vi "GetPen.vi"(8 "error in (no error)":errorcluster, 11 "Pen in":refnum<class "Pen.lvclass">) -> (0 "error out":errorcluster, 2 "Pen":T1, 3 "Pen out":refnum<class "Pen.lvclass">)   [LabVIEW 2021, in "Picture2D.lvlib" / "Pen.lvclass"]
uses:
  Pen.lvclass
  Pen.lvclass/Pen.ctl
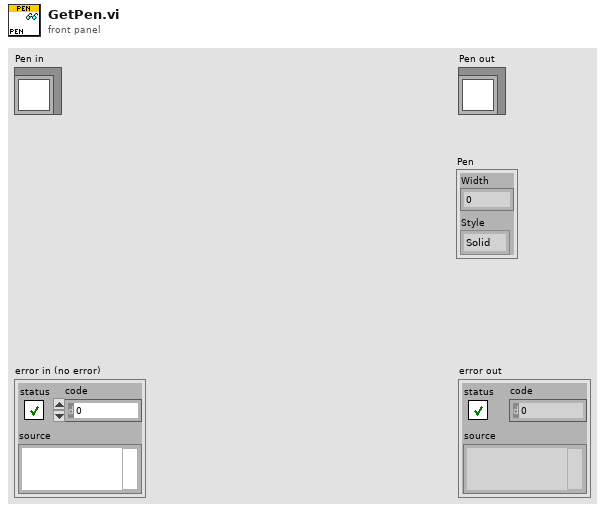
[diagram p1: front panel]
types:
  T1 = cluster{"Width":u16, "Style":enum32{"Solid", "Dash", "Dot", "DashDot", "DashDotDot"}}
  T2 = enum32{"Solid", "Dash", "Dot", "DashDot", "DashDotDot"}
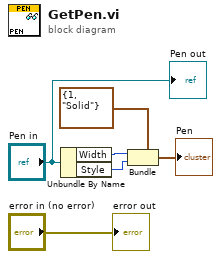
[diagram p0: block diagram]
diagram:
  n1 = Unbundle By Name("Pen in") -> ("Width"=w3:u16, "Style"=w2:T2)
  n2 = Bundle(cluster=T1 {"Width"=1, "Style"=enum."Solid"} ("pen"), "Width"=w3, "Style"=w2) -> (→"Pen":T1)
  "error out" <- "error in (no error)"
  "Pen out" <- "Pen in"
